vi "Submission from Result.vi"(8 "error in (no error)":errorcluster, 11 "Statement In":refnum<class "SQL Statement.lvclass">) -> (0 "error out":errorcluster, 2 "Submission":refnum<class "Submission.lvclass">, 3 "Statement":refnum<class "SQL Statement.lvclass">)   [LabVIEW 2020, in "Summer of LabVIEW.lvlib" / "Submission DB.lvclass"]
uses:
  Submission DB.lvclass
  <vilib>/drjdpowell/SQLite Library/SQL Statement/SQL Statement.lvclass
  Submission/Submission.lvclass
  Submission/Submission Data.ctl
  SoL Scoring/Score.ctl
  SoL Scoring/Score Entry.ctl
  <vilib>/drjdpowell/SQLite Library/SQL Statement/SQL Statement.lvclass/SQL Statement.ctl
  <vilib>/drjdpowell/SQLite Library/SQL Statement/Column I64.vi
  <vilib>/drjdpowell/SQLite Library/SQL Statement/Column String.vi
  Submission DB.lvclass/Submission DB.ctl
  SoL Scoring/SoL Scoring.lvlib
  <vilib>/IlluminatedG/lv-web-crypto/lv-json/JSON/JSON.lvlib
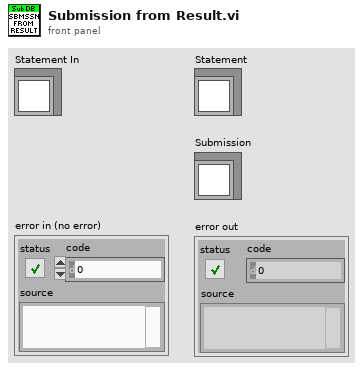
[diagram p1: front panel]
types:
  T1 = typedef "SoL Scoring.lvlib/Score.ctl" = cluster{"Overall":dbl, "Categories":T2[]}
  T2 = typedef "SoL Scoring.lvlib/Score Entry.ctl" = cluster{"Category":string, "Value":dbl}
  T3 = typedef "Summer of LabVIEW.lvlib/Submission.lvclass/Submission Data.ctl" = cluster{"ID":i64, "User ID":i64, "Challenge ID":i64, "Submitted":timestamp, "Score":T1, "Tested":bool, "Test Timestamp":timestamp, "Test Summary":string, "Approved for Test":bool, "Approver ID":i64, "Testing":bool}
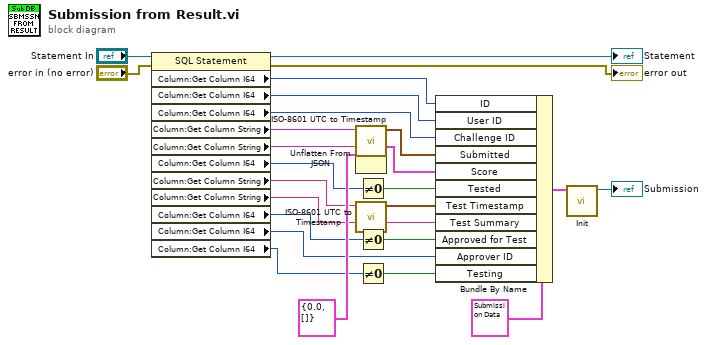
[diagram p0: block diagram]
diagram:
  n1 = property class="SQL Statement"(reference="Statement In", error in="error in (no error)") -> (reference out=→"Statement":refnum<class "SQL Statement.lvclass">, error out=→"error out":errorcluster, "Column:Get Column I64"=w24:i64, "Column:Get Column I64"=w23:i64, "Column:Get Column I64"=w22:i64, "Column:Get Column String"=w21:string, "Column:Get Column String"=w19:string, "Column:Get Column I64"=w16:i64, "Column:Get Column String"=w13:string, "Column:Get Column String"=w12:string, "Column:Get Column I64"=w10:i64, "Column:Get Column I64"=w9:i64, "Column:Get Column I64"=w2:i64)
  n2 = call <vilib>:"ISO-8601 UTC to Timestamp.vi"("ISO-8601"=w21) -> ("time stamp"=w20:timestamp)  [unwired: 9 in, 1 out]
  n3 = Unflatten From JSON(JSON string=w19, type and defaults=T1 {"Overall"=0.0, "Categories"=[]} ("Score")) -> (value=w17:T1)  [unwired: 5 in, 1 out]
  n4 = call <vilib>:"ISO-8601 UTC to Timestamp.vi"("ISO-8601"=w13) -> ("time stamp"=w14:timestamp)  [unwired: 9 in, 1 out]
  n5 = Not Equal To 0?(x=w16) -> (x != 0?=w15:bool)
  n6 = Not Equal To 0?(x=w10) -> (x != 0?=w11:bool)
  n7 = Not Equal To 0?(x=w2) -> (x != 0?=w1:bool)
  n8 = Bundle By Name(cluster=T3 {"ID"=0, "User ID"=0, "Challenge ID"=0, "Submitted"=timestamp(0 s since 1904-01-01), "Score"={"Overall"=0.0, "Categories"=[]}, "Tested"=FALSE, "Test Timestamp"=timestamp(0 s since 1904-01-01), "Test Summary"="", "Approved for Test"=FALSE, "Approver ID"=0, "Testing"=FALSE} ("Submission Data"), "ID"=w24, "User ID"=w23, "Challenge ID"=w22, "Submitted"=w20, "Score"=w17, "Tested"=w15, "Test Timestamp"=w14, "Test Summary"=w12, "Approved for Test"=w11, "Approver ID"=w9, "Testing"=w1) -> (w8:T3)
  n9 = call "Init.vi"("Submission Data"=w8) -> ("Submission out"=→"Submission":refnum<class "Submission.lvclass">)  [unwired: 9 in, 1 out]
